vi "Connector0 Analog Input.vi"() -> (0 "Packets":u64[](array[numeric]))   [LabVIEW 2010]
uses:
  <vilib>/eio/EIONode/EIONode.xnode
  <vilib>/rvi/eio/nirviEIOImplementation/nirviEIOImplementation.xnode
  <vilib>/rvi/eio/common/nirviEmuClasses.ctl
  <vilib>/rvi/eio/common/nirviEmuTemplateMethod_noerrors.vi
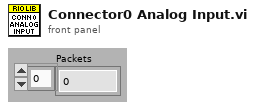
[diagram p1: front panel]
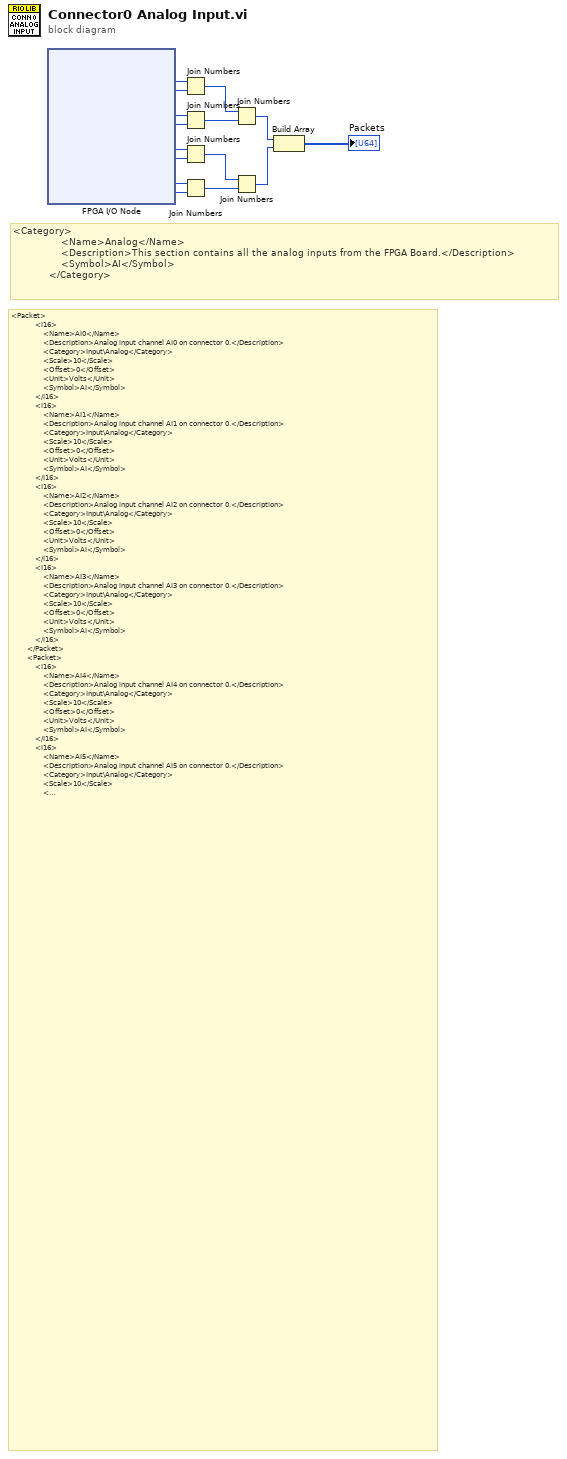
[diagram p0: block diagram]
diagram:
  # "<Category>\n                <Name>Analog</Name>\n                <Description>This section contains all the analog inputs from the FPGA Board.</Description>\n                <Symbol>AI</Symbol>\n            </Category>"
  # "<Packet>\n            <I16>\n                <Name>AI0</Name>\n                <Description>Analog input channel AI0 on connector 0.</Description>\n                <Category>Input\\Analog</Category>\n                <Scale>10</Scale>\n                <Offset>0</Offset>\n                <Unit>Volts</Unit>\n                <Symbol>AI</Symbol>\n            </I16>\n            <I16>\n                <Name>AI1</Name>\n                <Description>Analog input channel AI1 on connector 0.</Description>\n                <Category>Input\\Analog</Category>\n                <Scale>10</Scale>\n                <Offset>0</Offset>\n                <Unit>Volts</Unit>\n                <Symbol>AI</Symbol>\n            </I16>\n            <I16>\n                <Name>AI2</Name>\n                <Description>Analog input channel AI2 on connector 0.</Description>\n                <Category>Input\\Analog</Category>\n                <Scale>10</Scale>\n                <Offset>0</Offset>\n                <Unit>Volts</Unit>\n                <Symbol>AI</Symbol>\n            </I16>\n            <I16>\n                <Name>AI3</Name>\n                <Description>Analog input channel AI3 on connector 0.</Description>\n                <Category>Input\\Analog</Category>\n                <Scale>10</Scale>\n                <Offset>0</Offset>\n                <Unit>Volts</Unit>\n                <Symbol>AI</Symbol>\n            </I16>\n        </Packet>\n        <Packet>\n            <I16>\n                <Name>AI4</Name>\n                <Description>Analog input channel AI4 on connector 0.</Description>\n                <Category>Input\\Analog</Category>\n                <Scale>10</Scale>\n                <Offset>0</Offset>\n                <Unit>Volts</Unit>\n                <Symbol>AI</Symbol>\n            </I16>\n            <I16>\n                <Name>AI5</Name>\n                <Description>Analog input channel AI5 on connector 0.</Description>\n                <Category>Input\\Analog</Category>\n                <Scale>10</Scale>\n                <Offset>0</Offset>\n                <Unit>Volts</Unit>\n                <Symbol>AI</Symbol>\n            </I16>\n            <I16>\n                <Name>AI6</Name>\n                <Description>Analog input channel AI6 on connector 0.</Description>\n                <Category>Input\\Analog</Category>\n                <Scale>10</Scale>\n                <Offset>0</Offset>\n                <Unit>Volts</Unit>\n                <Symbol>AI</Symbol>\n            </I16>\n            <I16>\n                <Name>AI7</Name>\n                <Description>Analog input channel AI7 on connector 0.</Description>\n                <Category>Input\\Analog</Category>\n                <Scale>10</Scale>\n                <Offset>0</Offset>\n                <Unit>Volts</Unit>\n                <Symbol>AI</Symbol>\n            </I16>\n        </Packet>"
  n1 = xnode "FPGA I/O Node"() -> ("Connector0/AI3"=w1:i16, "Connector0/AI2"=w2:i16, "Connector0/AI1"=w3:i16, "Connector0/AI0"=w4:i16, "Connector0/AI7"=w5:i16, "Connector0/AI6"=w6:i16, "Connector0/AI5"=w7:i16, "Connector0/AI4"=w8:i16)  [unwired: 8 in, 8 out]
  n2 = Join Numbers(hi=w1, lo=w2) -> ((hi.lo)=w10:u32)
  n3 = Join Numbers(hi=w3, lo=w4) -> ((hi.lo)=w9:u32)
  n4 = Join Numbers(hi=w5, lo=w6) -> ((hi.lo)=w12:u32)
  n5 = Join Numbers(hi=w7, lo=w8) -> ((hi.lo)=w11:u32)
  n6 = Join Numbers(hi=w10, lo=w9) -> ((hi.lo)=w15:u64)
  n7 = Join Numbers(hi=w12, lo=w11) -> ((hi.lo)=w14:u64)
  n8 = Build Array(w15, w14) -> (→"Packets":u64[])
